vi "extract xyz segment with cursors.vi"(6 "sample rate":dbl, 8 "Zmag trajectory":waveform(dbl) caption="元素", 9 "cursor pos":dbl, 10 "data":waveform(dbl)[](array[waveform]), 11 "cursor length":dbl) -> (0 "Z":dbl[](array[numeric]), 1 "Y":dbl[](array[numeric]), 2 "X":dbl[](array[numeric]), 3 "xy cluster":cluster{dbl[], dbl[]}, 4 "Z mag":dbl[](array[numeric]))   [LabVIEW 2017]
doc: "本VI 用于将双游标选定的区域包含的xy 数据提取出来，然后化成xy方向的图，用来观察横向布朗运动的情况。\n本VI 可用于挑选比较好的参考球（漂移小），以后如果有需要还可以在旋转过程中测量，判断圆心之类的。\n需要注意的是，本VI是以单个球输入为假设来设计的，也就是说，输入的数据应该是一个组名称下的一组xyz等数据，而不是一个组名称下的多个xyz组数据。"
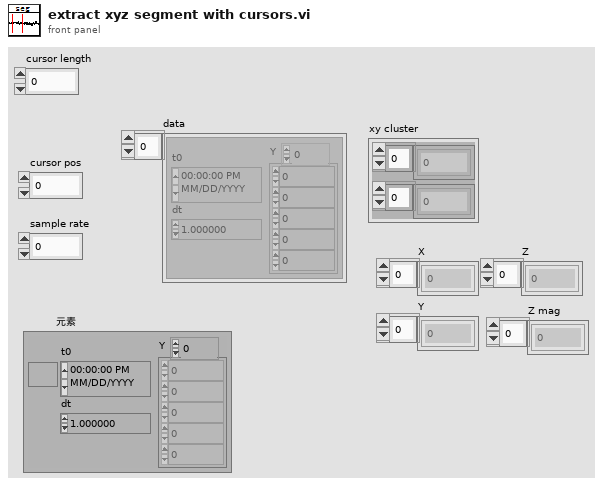
[diagram p1: front panel]
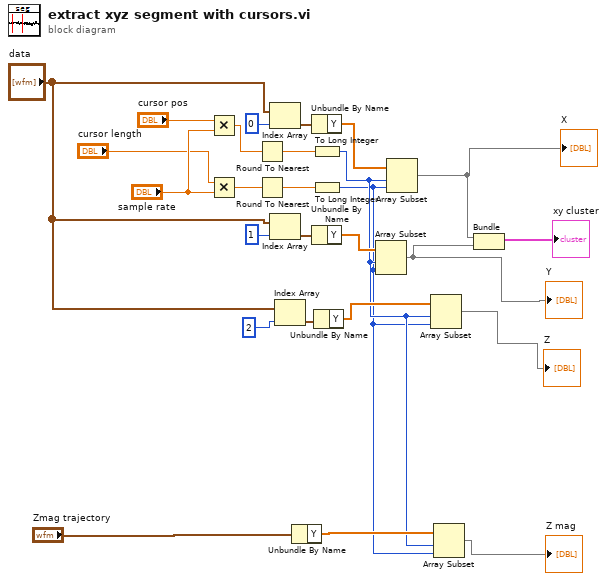
[diagram p0: block diagram]
diagram:
  n1 = Multiply(x="cursor pos", y="sample rate") -> (x*y=w18:dbl)
  n2 = Multiply(x="cursor length", y="sample rate") -> (x*y=w23:dbl)
  n3 = Round To Nearest(number=w18) -> (nearest integer value=w19:dbl)
  n4 = Round To Nearest(number=w23) -> (nearest integer value=w22:dbl)
  n5 = Index Array(array="data", index=0 ("索引")) -> (element=w15:waveform(dbl))
  n6 = Index Array(array="data", index=1 ("索引")) -> (element=w16:waveform(dbl))
  n7 = Index Array(array="data", index=2 ("索引")) -> (element=w10:waveform(dbl))
  n8 = Unbundle By Name("Zmag trajectory") -> ("Y"=w4:dbl[])
  n9 = Unbundle By Name(w15) -> ("Y"=w20:dbl[])
  n10 = To Long Integer(number=w19) -> (32bit integer=w3:i32)
  n11 = To Long Integer(number=w22) -> (32bit integer=w2:i32)
  n12 = Unbundle By Name(w16) -> ("Y"=w21:dbl[])
  n13 = Unbundle By Name(w10) -> ("Y"=w9:dbl[])
  n14 = Array Subset(array=w21, index=w3, length=w2) -> (w7:dbl[])
  "Y" <- w7
  n15 = Array Subset(array=w20, index=w3, length=w2) -> (w8:dbl[])
  "X" <- w8
  n16 = Array Subset(array=w9, index=w3, length=w2) -> (→"Z":dbl[])
  n17 = Array Subset(array=w4, index=w3, length=w2) -> (→"Z mag":dbl[])
  n18 = Bundle(w8, w7) -> (→"xy cluster":cluster{dbl[], dbl[]})  [unwired: 1 in]
